vi "NGTS_Read Taglist Files.vi"(0 "Tag Set Directory":path=path "c:/ni-rt/startup/Config_Files", 1 "Get-Load Action":T1, 11 "error in":errorcluster) -> (3 "Memory Tags Properties Table":string[][](array[string]), 4 "AI Channels Properties Table":string[][](array[string]), 6 "AO Channels Properties Table":string[][](array[string]), 8 "DI Channels Properties Table":string[][](array[string]), 10 "DO Channels Properties Table":string[][](array[string]), 14 "Ext Instruments Channels Properties Table":string[][](array[string]), 15 "error out":errorcluster)   [LabVIEW 2018]
doc: "Reads in the 7 Tag definition files from the indicated directory. These files are string formatted tab delimited text spreadsheet files. The Memory and Output files should all have Expressions (formulas) in the last column.\n\n Memory_Tags.txt\n Analog Input_Tags.txt\n Thermocouples_Tags.txt\n Analog Output_Tags.txt\n Digital Input_Tags.txt\n Digital Output_Tags.txt\n Ext Instruments_Tags.txt\n\nCurrently the Thermocouple file is concatenated with the Analog Input table.\n2007_12 Mike Ashe\nmichael.ashe@imaginatics.net\nCell: 860-961-0876\n2008_02 updated ROH"
uses:
  Controls/ENUM Get-Load Action.ctl
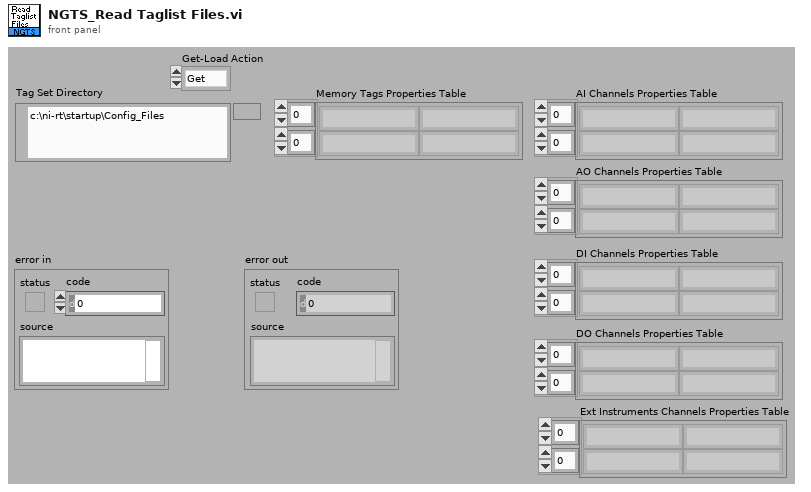
[diagram p1: front panel]
types:
  T1 = typedef "ENUM Get-Load Action.ctl" = enum16{"Get", "Load"}
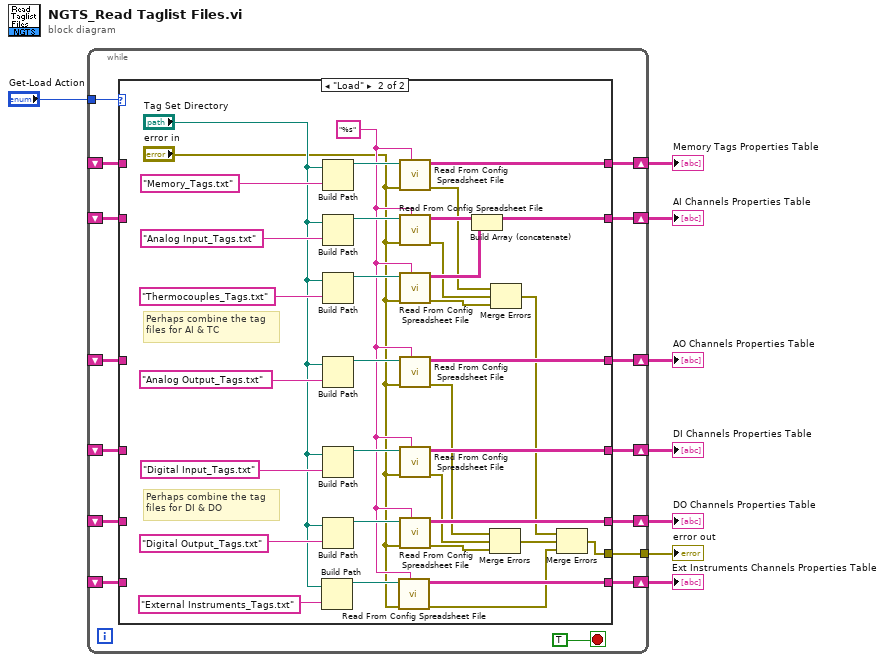
[diagram p0: block diagram]
diagram:
  n1 = while {
    tunnel: [w17] -> w2
    shift-right: [w19] -> w4
    shift-left: _ -> [w14]
    tunnel: "Get-Load Action" -> [w15]
    shift-right: [w22] -> w7
    shift-left: _ -> [w13]
    shift-right: [w23] -> w8
    shift-left: _ -> [w12]
    shift-right: [w20] -> w5
    shift-left: _ -> [w11]
    shift-right: [w21] -> w6
    shift-left: _ -> [w10]
    shift-right: [w18] -> w3
    shift-left: _ -> [w9]
    stop <- TRUE stop-if-true
    n2 = case shown="\"Load\"" w15 {
      tunnel: [w27 w64] -> w23
      tunnel: [w28 w51] -> w22
      tunnel: [w25 w50] -> w21
      tunnel: [w26 w49] -> w20
      tunnel: [w29 w46] -> w19
      tunnel: [w24 w45] -> w18
      tunnel: [_ w32] -> w17
      tunnel: w14 -> [w29 _]
      tunnel: w13 -> [w28 _]
      tunnel: w12 -> [w27 _]
      tunnel: w11 -> [w26 _]
      tunnel: w10 -> [w25 _]
      tunnel: w9 -> [w24 _]
      frame "Get", Default {
      }
      frame "Load" {
        w41 = "%s" ("format (%s)")
        # "Perhaps combine the tag\nfiles for DI & DO"
        # "Perhaps combine the tag\nfiles for AI & TC"
        n3 = Build Path(base path="Tag Set Directory", name or relative path="External Instruments_Tags.txt") -> (appended path=w43:path)
        n4 = Build Path(base path="Tag Set Directory", name or relative path="Memory_Tags.txt") -> (appended path=w48:path)
        n5 = Build Path(base path="Tag Set Directory", name or relative path="Analog Input_Tags.txt") -> (appended path=w62:path)
        n6 = Build Path(base path="Tag Set Directory", name or relative path="Thermocouples_Tags.txt") -> (appended path=w55:path)
        n7 = Build Path(base path="Tag Set Directory", name or relative path="Analog Output_Tags.txt") -> (appended path=w61:path)
        n8 = Build Path(base path="Tag Set Directory", name or relative path="Digital Input_Tags.txt") -> (appended path=w60:path)
        n9 = Build Path(base path="Tag Set Directory", name or relative path="Digital Output_Tags.txt") -> (appended path=w57:path)
        n10 = call "Read From Config Spreadsheet File.vi"("format (%s)"=w41, "error in"="error in", "file path (dialog if empty)"=w43) -> ("error out"=w30:errorcluster, "all rows"=w45:string[][])  [unwired: 6 in, 1 out]
        n11 = call "Read From Config Spreadsheet File.vi"("format (%s)"=w41, "error in"="error in", "file path (dialog if empty)"=w48) -> ("error out"=w40:errorcluster, "all rows"=w46:string[][])  [unwired: 6 in, 1 out]
        n12 = call "Read From Config Spreadsheet File.vi"("format (%s)"=w41, "error in"="error in", "file path (dialog if empty)"=w62) -> ("error out"=w39:errorcluster, "all rows"=w52:string[][])  [unwired: 6 in, 1 out]
        n13 = call "Read From Config Spreadsheet File.vi"("format (%s)"=w41, "error in"="error in", "file path (dialog if empty)"=w55) -> ("error out"=w38:errorcluster, "all rows"=w53:string[][])  [unwired: 6 in, 1 out]
        n14 = call "Read From Config Spreadsheet File.vi"("format (%s)"=w41, "error in"="error in", "file path (dialog if empty)"=w61) -> ("error out"=w37:errorcluster, "all rows"=w64:string[][])  [unwired: 6 in, 1 out]
        n15 = call "Read From Config Spreadsheet File.vi"("format (%s)"=w41, "error in"="error in", "file path (dialog if empty)"=w60) -> ("error out"=w36:errorcluster, "all rows"=w49:string[][])  [unwired: 6 in, 1 out]
        n16 = call "Read From Config Spreadsheet File.vi"("format (%s)"=w41, "error in"="error in", "file path (dialog if empty)"=w57) -> ("error out"=w35:errorcluster, "all rows"=w50:string[][])  [unwired: 6 in, 1 out]
        n17 = Build Array (concatenate)(w52, w53) -> (w51:string[][])
        n18 = Merge Errors(w37, w36, w35) -> (w34:errorcluster)
        n19 = Merge Errors(w40, w39, w38) -> (w33:errorcluster)
        n20 = Merge Errors(w33, w34, w30) -> (w32:errorcluster)
      }
    }
  }
  "AI Channels Properties Table" <- w7
  "AO Channels Properties Table" <- w8
  "error out" <- w2
  "DI Channels Properties Table" <- w5
  "DO Channels Properties Table" <- w6
  "Memory Tags Properties Table" <- w4
  "Ext Instruments Channels Properties Table" <- w3
